vi "Analog_Output_1.vi"() -> ()   [LabVIEW 2019]
uses:
  <vilib>/DAQmx/write.llb/DAQmx Write (Analog Wfm 1Chan NSamp).vi
  <vilib>/DAQmx/create/channels.llb/DAQmx Create Channel (AO-Voltage-Basic).vi
  <vilib>/DAQmx/configure/timing.llb/DAQmx Timing (Use Waveform).vi
  <vilib>/DAQmx/configure/trigger.llb/DAQmx Start Trigger (Digital Edge).vi
  <vilib>/DAQmx/miscellaneous.llb/DAQmx Fill In Error Info.vi
  <vilib>/measure/NI_MABase.lvlib
panel:
  in  "source":tag caption="소스"
  in  "physical channels":tag caption="물리적 채널"
  out "웨이브폼 그래프":waveform(dbl)(graph)
  in  "amplitude":dbl=1.0 caption="진폭" format="%0.2p"
  in  "frequency":dbl=10.0 caption="주파수" format="%0.2p"
  in  "sampling info":cluster{"Fs":dbl, "#s":dbl}={"Fs"=1000.0, "#s"=1000.0} caption="샘플링 정보" {"Fs" format="%.2p"}
  in  "edge":i32(ring)=10280 caption="에지" items=["상승"=10280, "하강"=10171]
  in  "정지버튼":bool
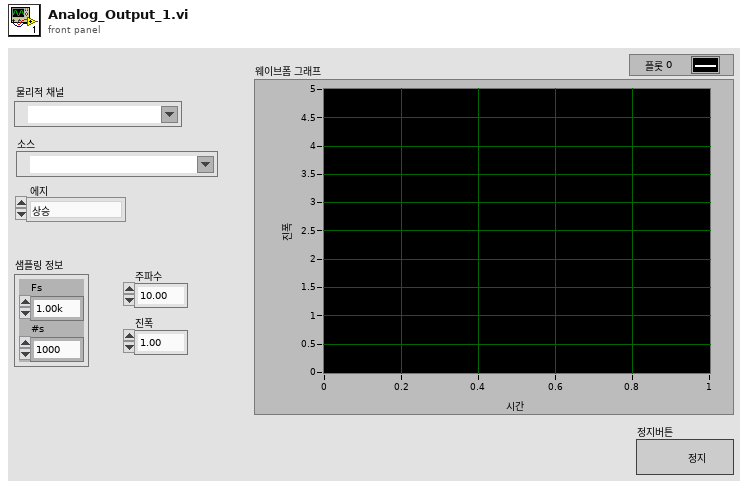
[diagram p1: front panel]
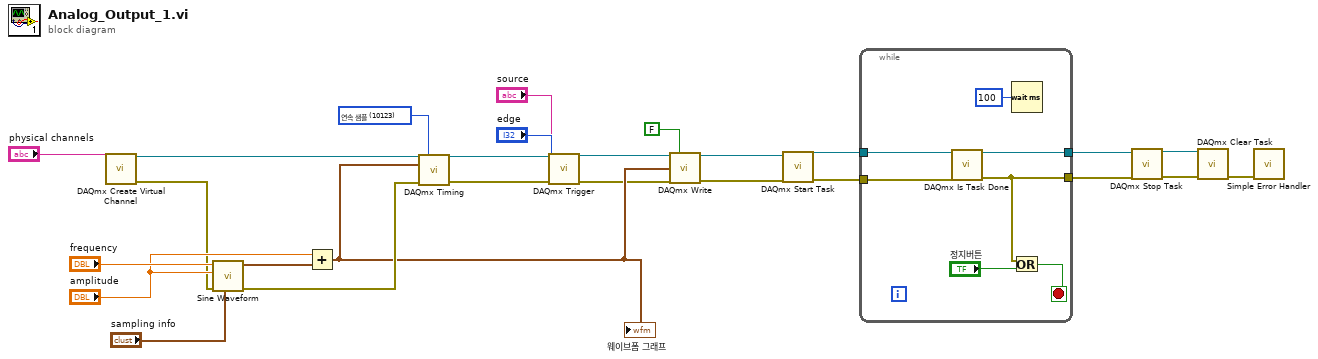
[diagram p0: block diagram]
diagram:
  w19 = 10123 items=["유한 샘플"=10178, "연속 샘플"=10123, "하드웨어 타이밍에 의한 단일 포인트"=12522] ("sample mode")
  n1 = call-poly <vilib>:"DAQmx Create Virtual Channel.vi"("physical channels"="physical channels") -> ("task out"=w10:refnum<k21>, "error out"=w11:errorcluster)  [unwired: 13 in]
  n2 = call <vilib>:"Sine Waveform.vi"("sampling info"="sampling info", "error in (no error)"=w11, "amplitude"="amplitude", "frequency"="frequency") -> ("error out"=w9:errorcluster, "signal out"=w13:waveform(dbl))  [unwired: 6 in]
  n3 = Add(x="amplitude", y=w13) -> (x+y=w8:waveform(dbl))
  "웨이브폼 그래프" <- w8
  n4 = call-poly <vilib>:"DAQmx Timing.vi"("task/channels in"=w10, "sample mode"=w19, "waveform"=w8, "error in"=w9) -> ("task out"=w17:refnum<k21>, "error out"=w16:errorcluster)  [unwired: 10 in]
  n5 = call-poly <vilib>:"DAQmx Trigger.vi"("task/channels in"=w17, "source"="source", "edge"="edge", "error in"=w16) -> ("task out"=w7:refnum<k21>, "error out"=w6:errorcluster)  [unwired: 10 in]
  n6 = call-poly <vilib>:"DAQmx Write.vi"("task/channels in"=w7, "auto start"=FALSE, "data"=w8, "error in"=w6) -> ("task out"=w4:refnum<k21>, "error out"=w5:errorcluster)  [unwired: 9 in, 1 out]
  n7 = call <vilib>:"DAQmx Start Task.vi"("task/channels in"=w4, "error in"=w5) -> ("task out"=w26:refnum<k21>, "error out"=w25:errorcluster)  [unwired: 12 in]
  n8 = while {
    tunnel: w26 -> [w33]
    tunnel: w25 -> [w32]
    tunnel: [w28] -> w24
    tunnel: [w29] -> w23
    stop <- w31 stop-if-true
    n9 = call <vilib>:"DAQmx Is Task Done.vi"("task/channels in"=w33, "error in"=w32) -> ("task out"=w28:refnum<k21>, "error out"=w29:errorcluster)  [unwired: 11 in, 1 out]
    n10 = Wait (ms)(milliseconds to wait=u32 100 ("대기 시간 (ms)")) -> ()  [unwired: 1 out]
    n11 = Or(x=w29, y="정지버튼") -> (x .or. y?=w31:bool)
  }
  n12 = call <vilib>:"DAQmx Stop Task.vi"("task/channels in"=w24, "error in"=w23) -> ("task out"=w22:refnum<k21>, "error out"=w21:errorcluster)  [unwired: 12 in]
  n13 = call <vilib>:"DAQmx Clear Task.vi"("task in"=w22, "error in"=w21) -> ("error out"=w20:errorcluster)  [unwired: 13 in]
  n14 = call <vilib>:"Simple Error Handler.vi"("error in (no error)"=w20) -> ()  [unwired: 4 in, 5 out]
